vi "camera decode.vi"(11 "Numeric":u32) -> (0 "command 2":string, 3 "command 1":string)   [LabVIEW 2021]
panel:
  out "Array 2":u8[](array[numeric])
  out "Array 1":u8[](array[numeric])
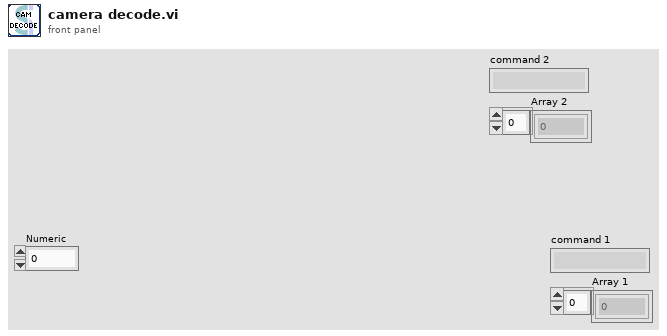
[diagram p1: front panel]
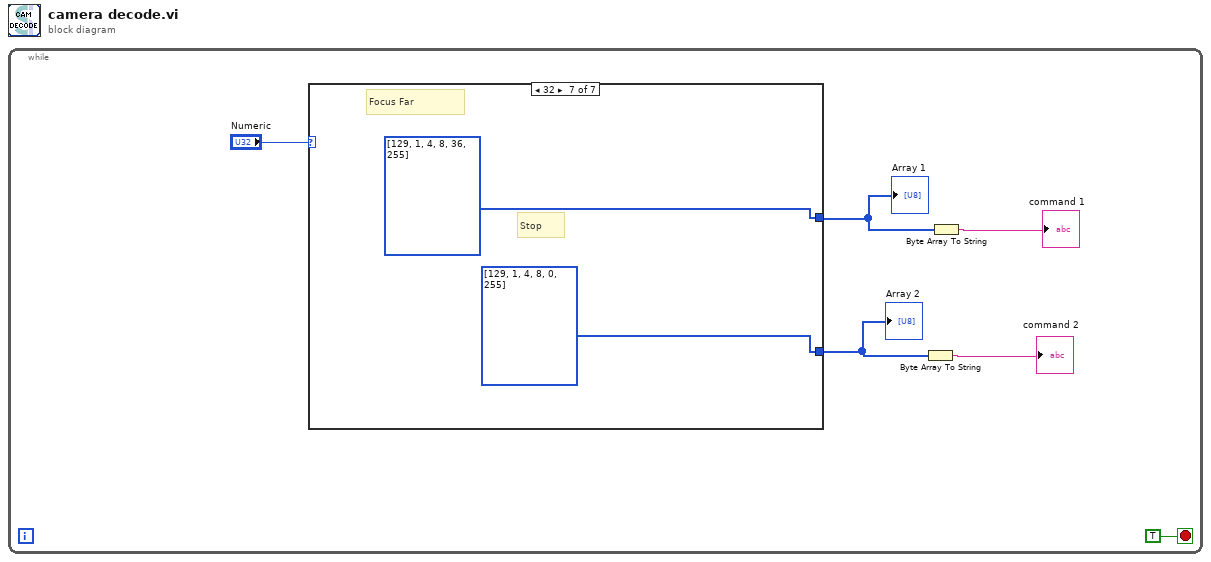
[diagram p0: block diagram]
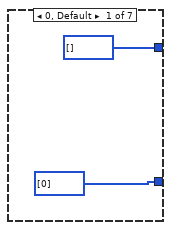
[diagram p2: hidden frame]
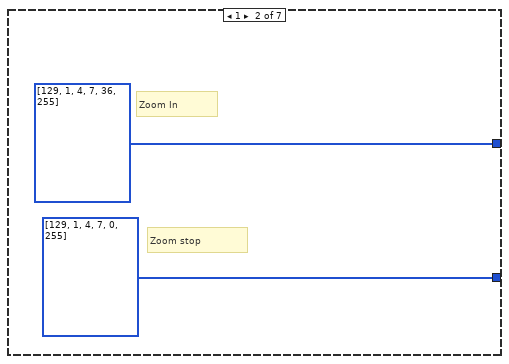
[diagram p3: hidden frame]
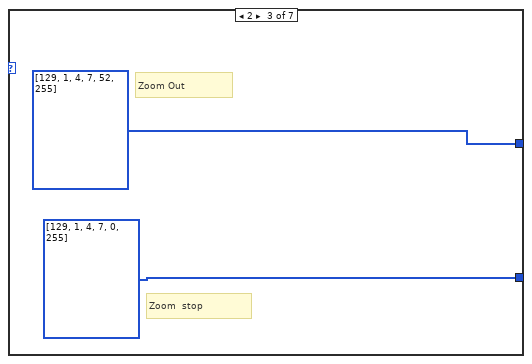
[diagram p4: hidden frame]
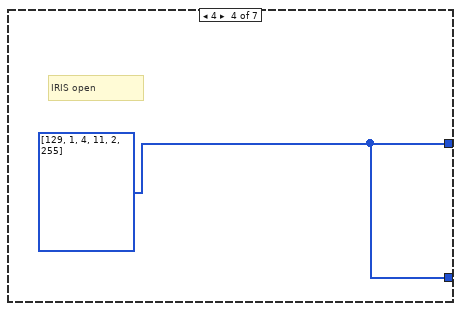
[diagram p5: hidden frame]
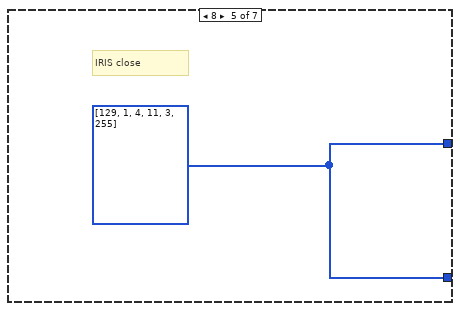
[diagram p6: hidden frame]
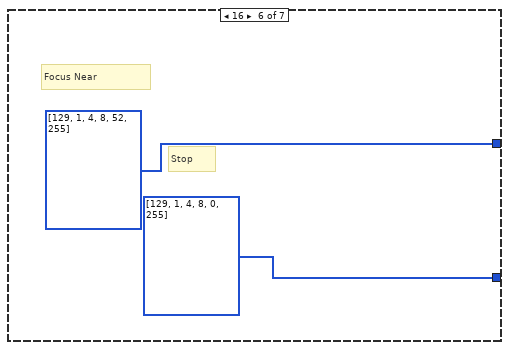
[diagram p7: hidden frame]
diagram:
  n1 = while {
    stop <- TRUE stop-if-true
    n2 = case shown="32" "Numeric" {
      tunnel: [u8[] [] u8[] [129, 1, 4, 7, 36, 255] u8[] [129, 1, 4, 7, 52, 255] w13 w14 u8[] [129, 1, 4, 8, 52, 255] u8[] [129, 1, 4, 8, 36, 255]] -> w3
      tunnel: [u8[] [0] u8[] [129, 1, 4, 7, 0, 255] u8[] [129, 1, 4, 7, 0, 255] w13 w14 u8[] [129, 1, 4, 8, 0, 255] u8[] [129, 1, 4, 8, 0, 255]] -> w1
      frame 0, Default {
      }
      frame 1 {
        # "Zoom stop"
        # "Zoom In"
      }
      frame 2 {
        # "Zoom  stop"
        # "Zoom Out"
      }
      frame 4 {
        w13 = u8[] [129, 1, 4, 11, 2, 255]
        # "IRIS open"
      }
      frame 8 {
        w14 = u8[] [129, 1, 4, 11, 3, 255]
        # "IRIS close"
      }
      frame 16 {
        # "Stop"
        # "Focus Near"
      }
      frame 32 {
        # "Stop"
        # "Focus Far"
      }
    }
    "Array 1" <- w3
    "Array 2" <- w1
    n3 = Byte Array To String(unsigned byte array=w1) -> (string=→"command 2":string)
    n4 = Byte Array To String(unsigned byte array=w3) -> (string=→"command 1":string)
  }
